vi "SingleSpectrum.vi"(0 "identifier out":string, 1 "Acquisition mode":u16(ring)=1 items=["Single spectrum", "Multiple spectra"], 2 "DPP Configuration":T1, 3 "Number of boards in chain":u8(slide)=1 scale=1.0..8.0, 4 "Boards to configure":u8(slide) scale=0.0..8.0, 6 "Start acq":bool, 7 "Stop":bool, 9 "Map points":u32=10, 11 "Time per spectrum [ms]":u32=10 max=1000000, 12 "reference":refnum<vi>, 13 "Acquisition time [s]":dbl=10.0 min=0.0009999999310821295 max=1000.0, 17 "Waveform Refnum":refnum<vi>, 18 "LastSpectra Refnum":refnum<vi>, 19 "SpectraPlot Refnum":refnum<vi>) -> (10 "Error code":i32, 14 "Acq. in progress":bool, 15 "Waveform Graph":dbl[][](graph))   [LabVIEW 2015]
uses:
  SingleSpectrumAcq.ctl
  GlobalParameters/SpectraData2.vi
  XGL_DPP.lvlib
panel:
  out "final time":u32
  out "live time":u32
  out "Init time":u32
  out "total_time":u32
  out "spectra to read":i64=1
  out "Statistics":dbl[][](array[numeric])
  out "adv stats":u64[][](array[numeric])
  out "spectra":u16[][](array[numeric])
  out "Library Initialized":bool
  in  "IP Address":string="10.96.0.110"
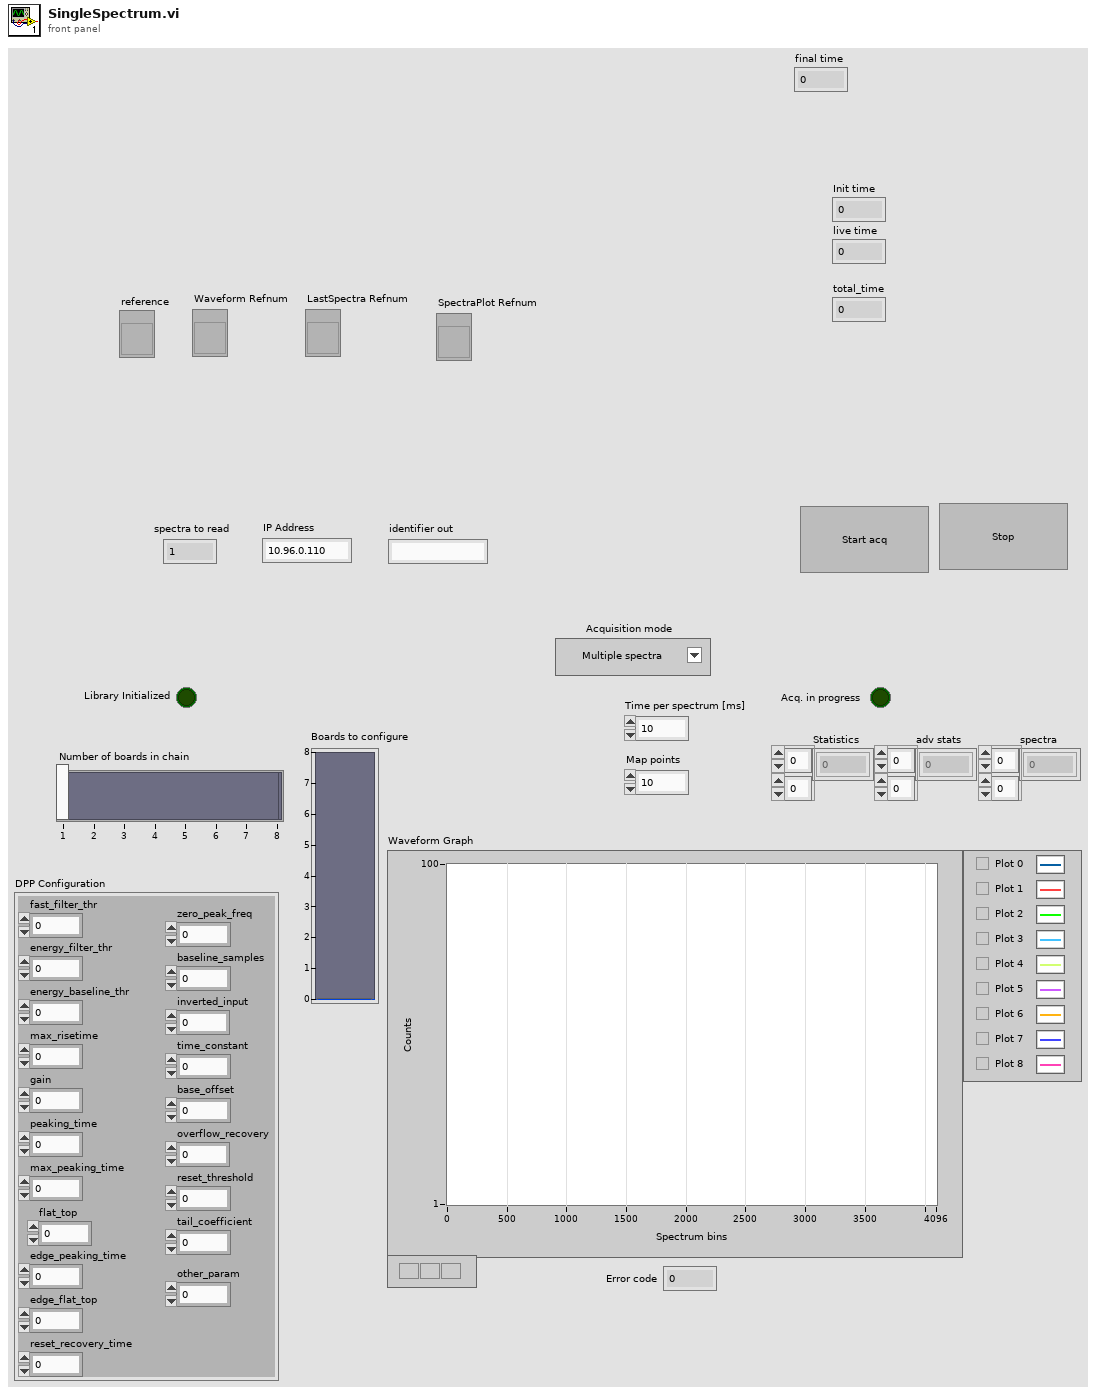
[diagram p1: front panel]
types:
  T1 = cluster{"reset_recovery_time":u32, "edge_peaking_time":u32, "flat_top":u32, "peaking_time":u32, "gain":dbl, "max_risetime":dbl, "fast_filter_thr":u32, "zero_peak_freq":dbl, "inverted_input":u8, "base_offset":u32, "reset_threshold":u32, "overflow_recovery":u32, "tail_coefficient":dbl, "energy_filter_thr":u32, "energy_baseline_thr":u32, "max_peaking_time":u32, "edge_flat_top":u32, "time_constant":dbl, "baseline_samples":u32, "other_param":u32}
  T2 = typedef "SingleSpectrumAcq.ctl" = enum16{"Stop", "Check downloaded spectra", "Get all data", "Read acq mode", "Send running/Get Data", "Clear", "Acquisition start", "Check Answer", "Wait Answer", "Start map"}
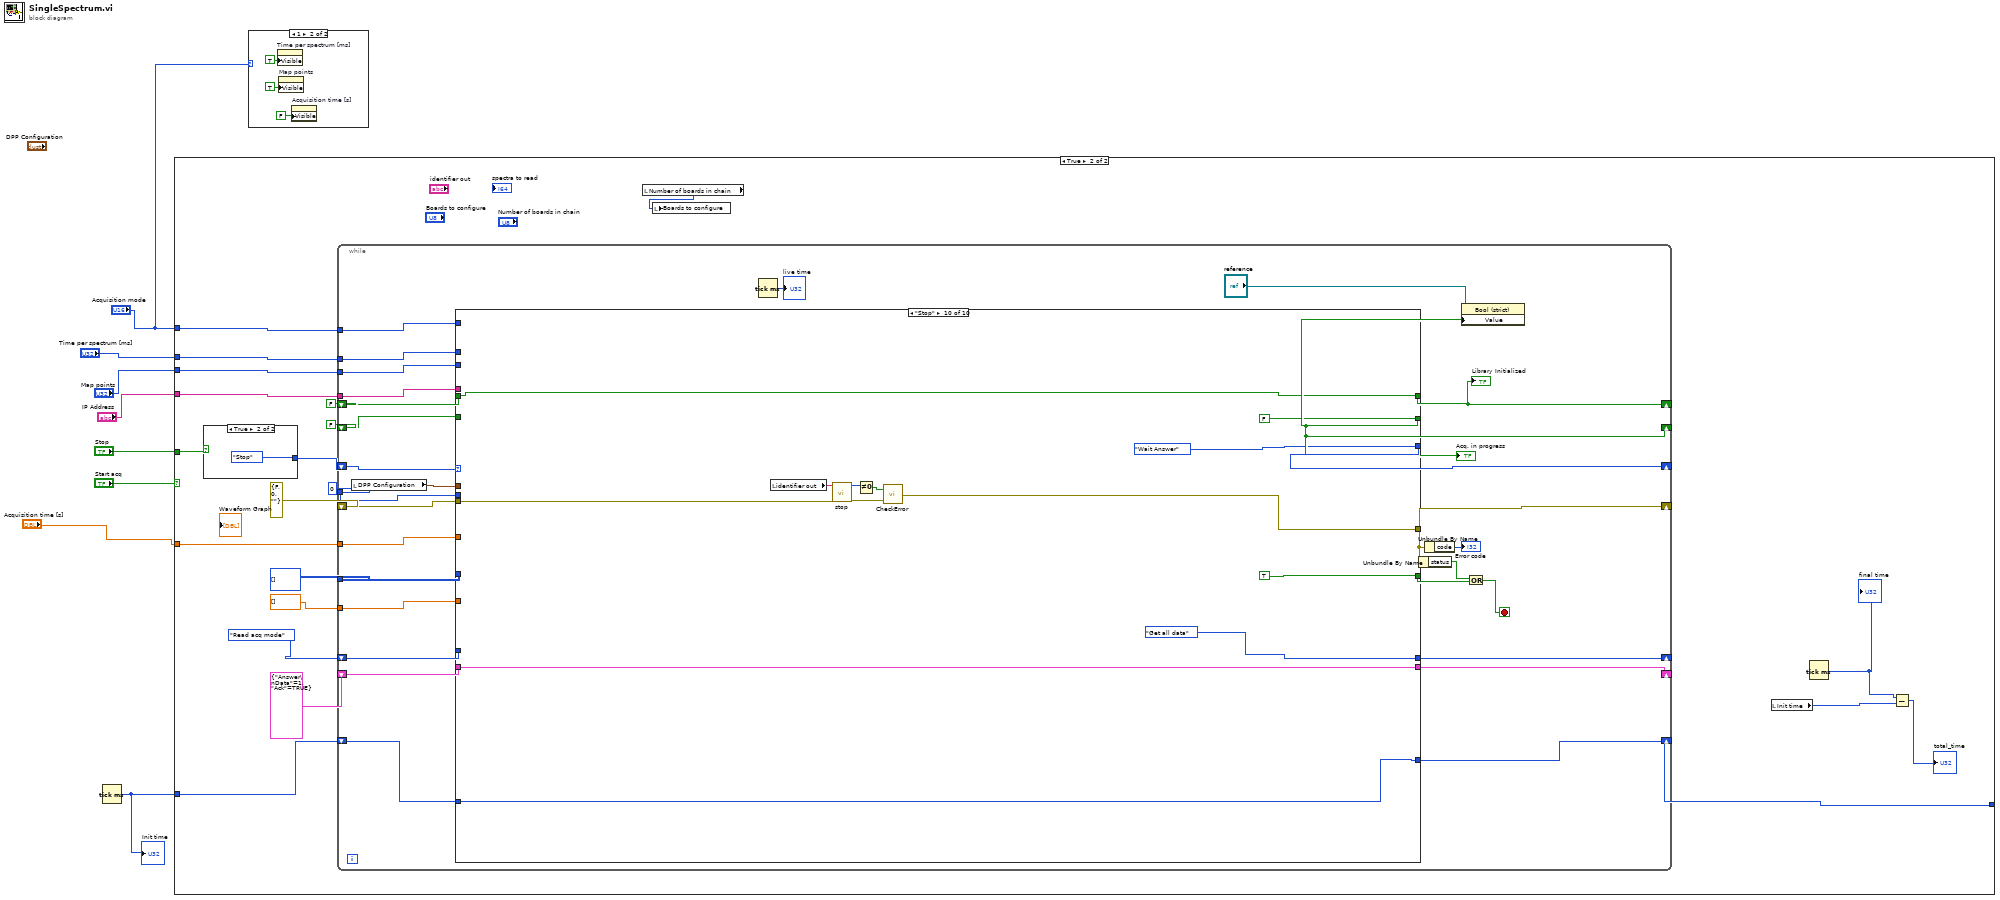
[diagram p0: block diagram]
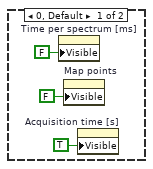
[diagram p2: hidden frame]
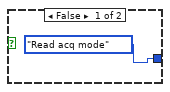
[diagram p4: hidden frame]
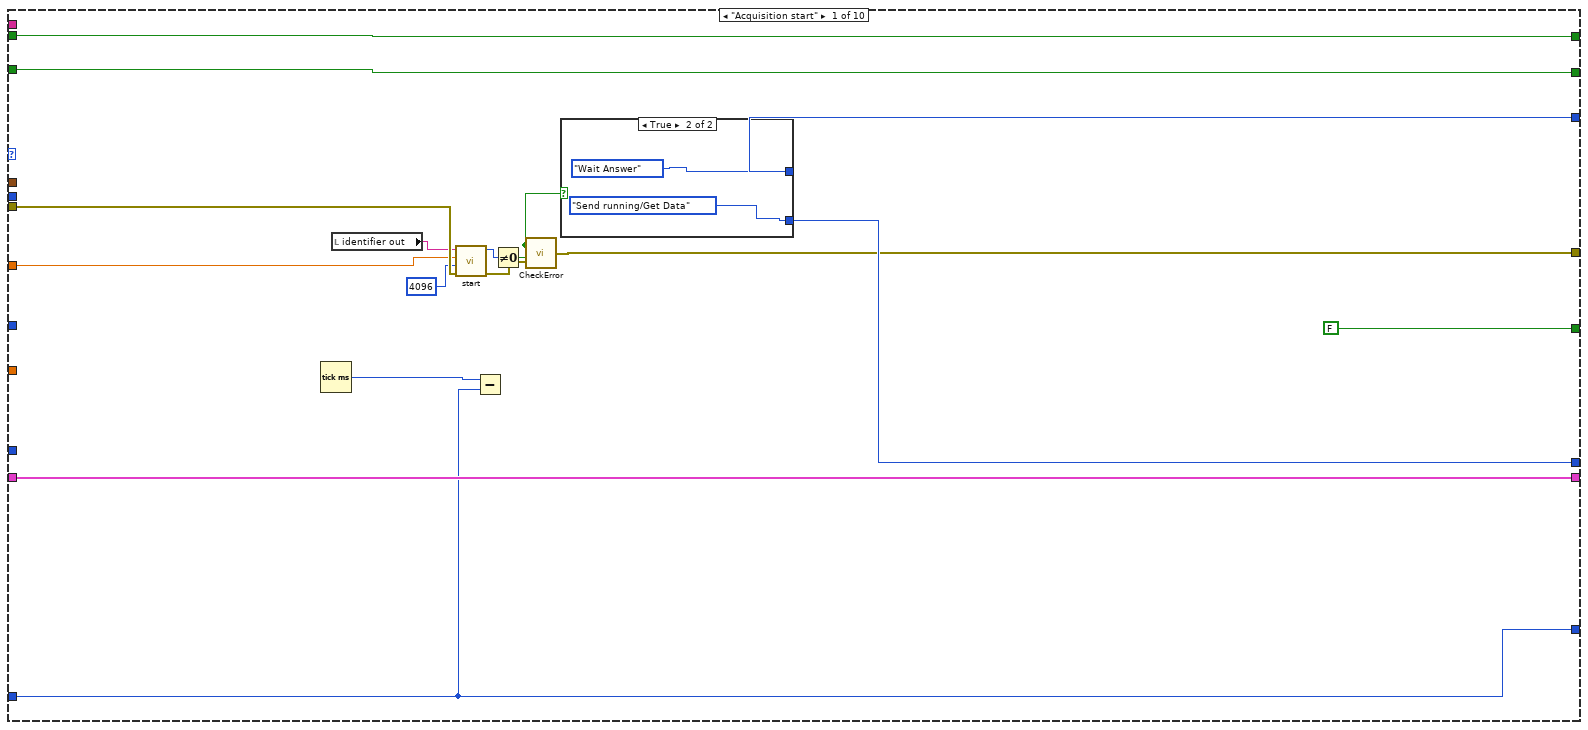
[diagram p5: hidden frame]
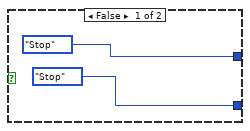
[diagram p6: hidden frame]
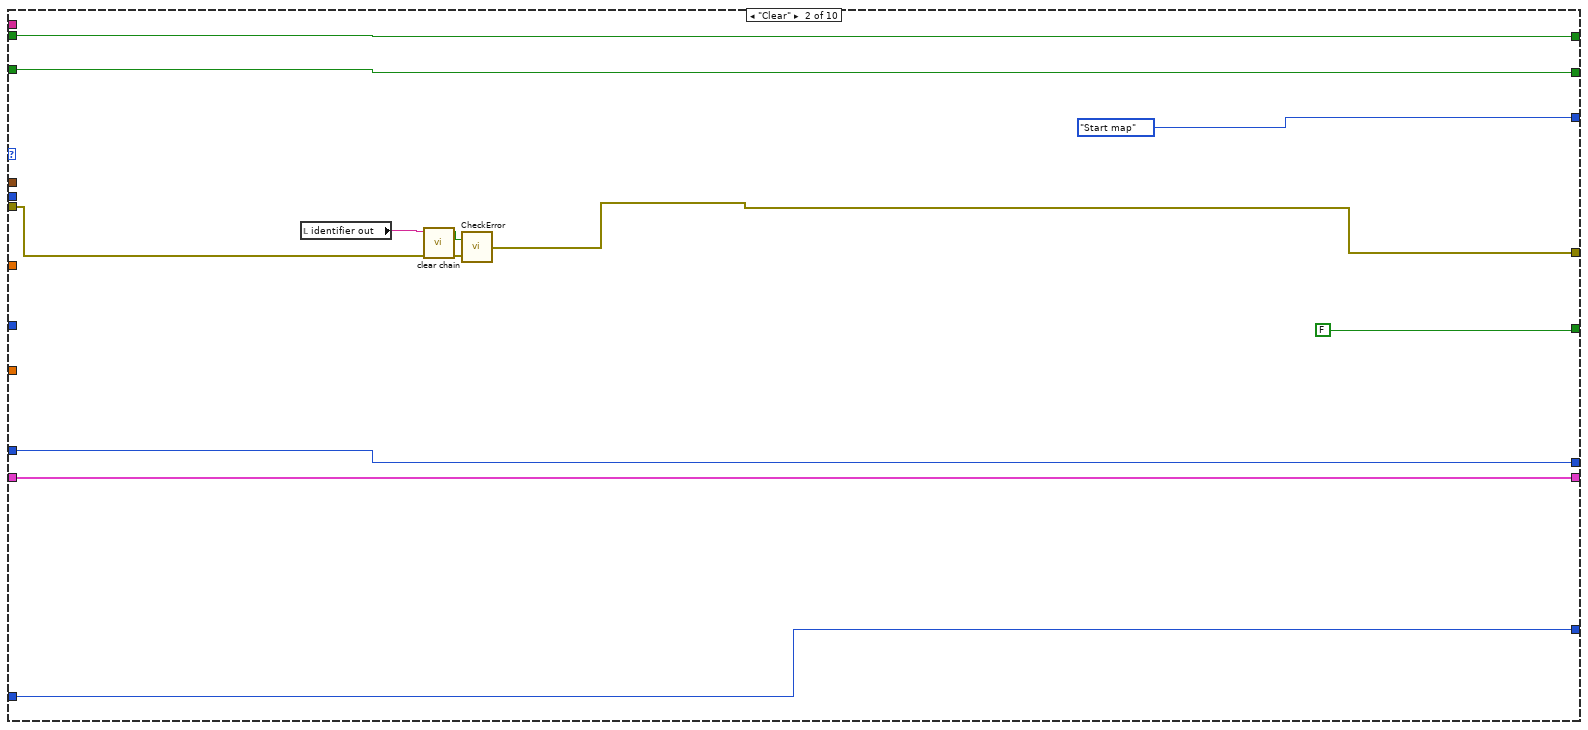
[diagram p7: hidden frame]
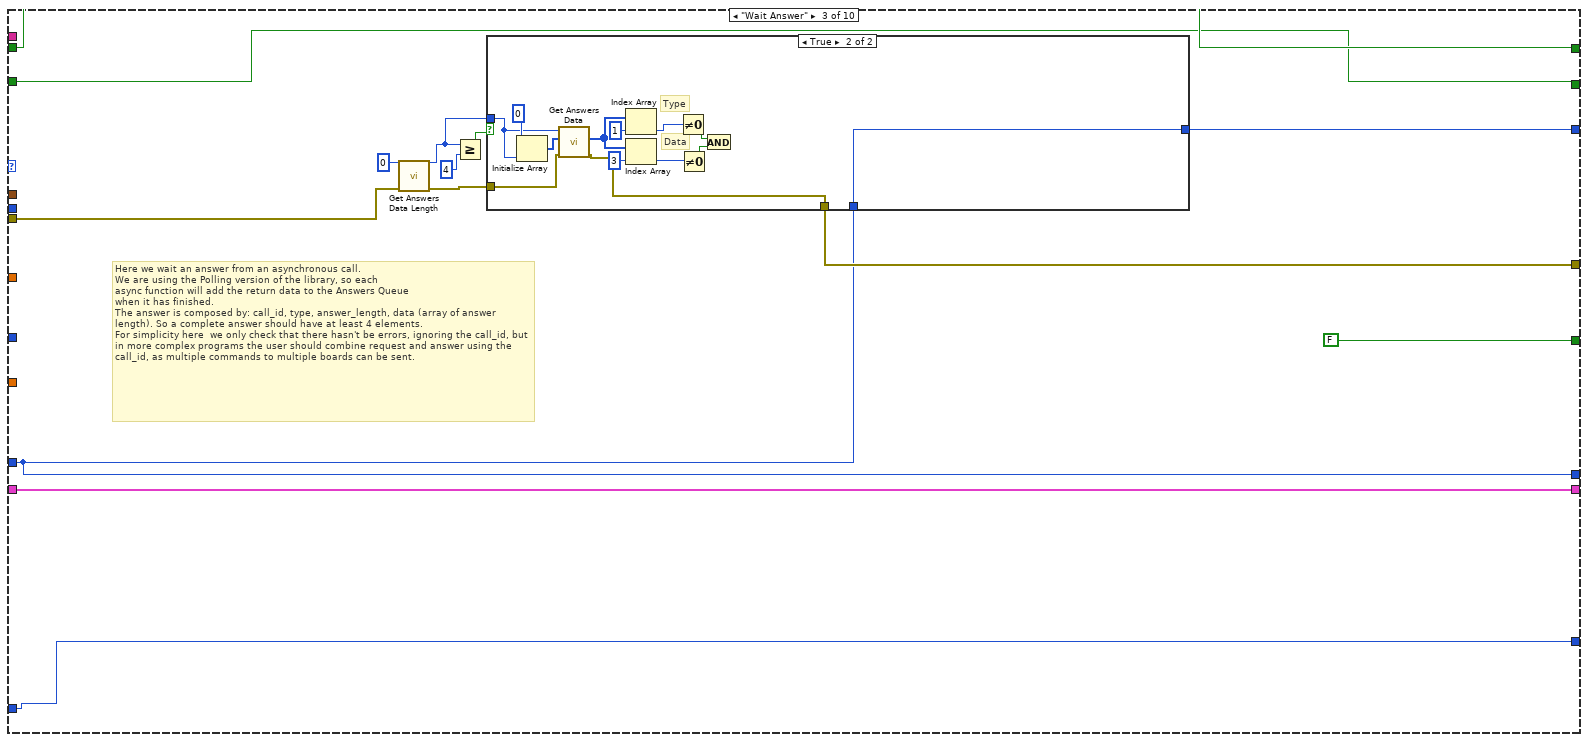
[diagram p8: hidden frame]
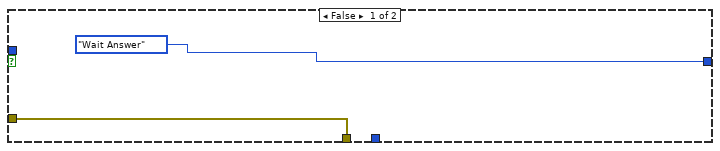
[diagram p9: hidden frame]
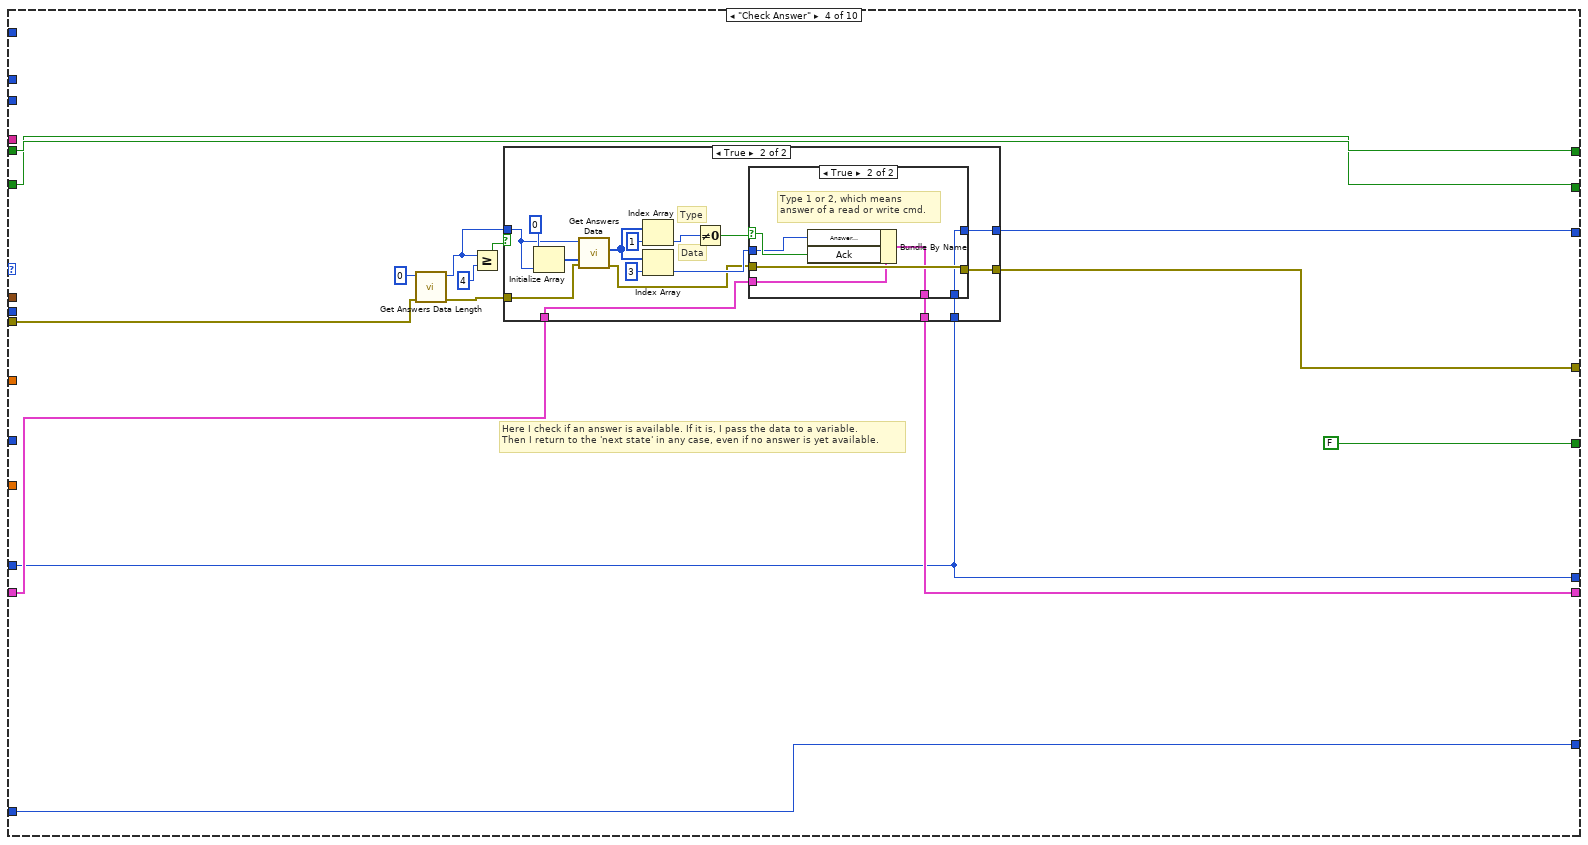
[diagram p10: hidden frame]
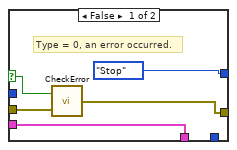
[diagram p12: hidden frame]
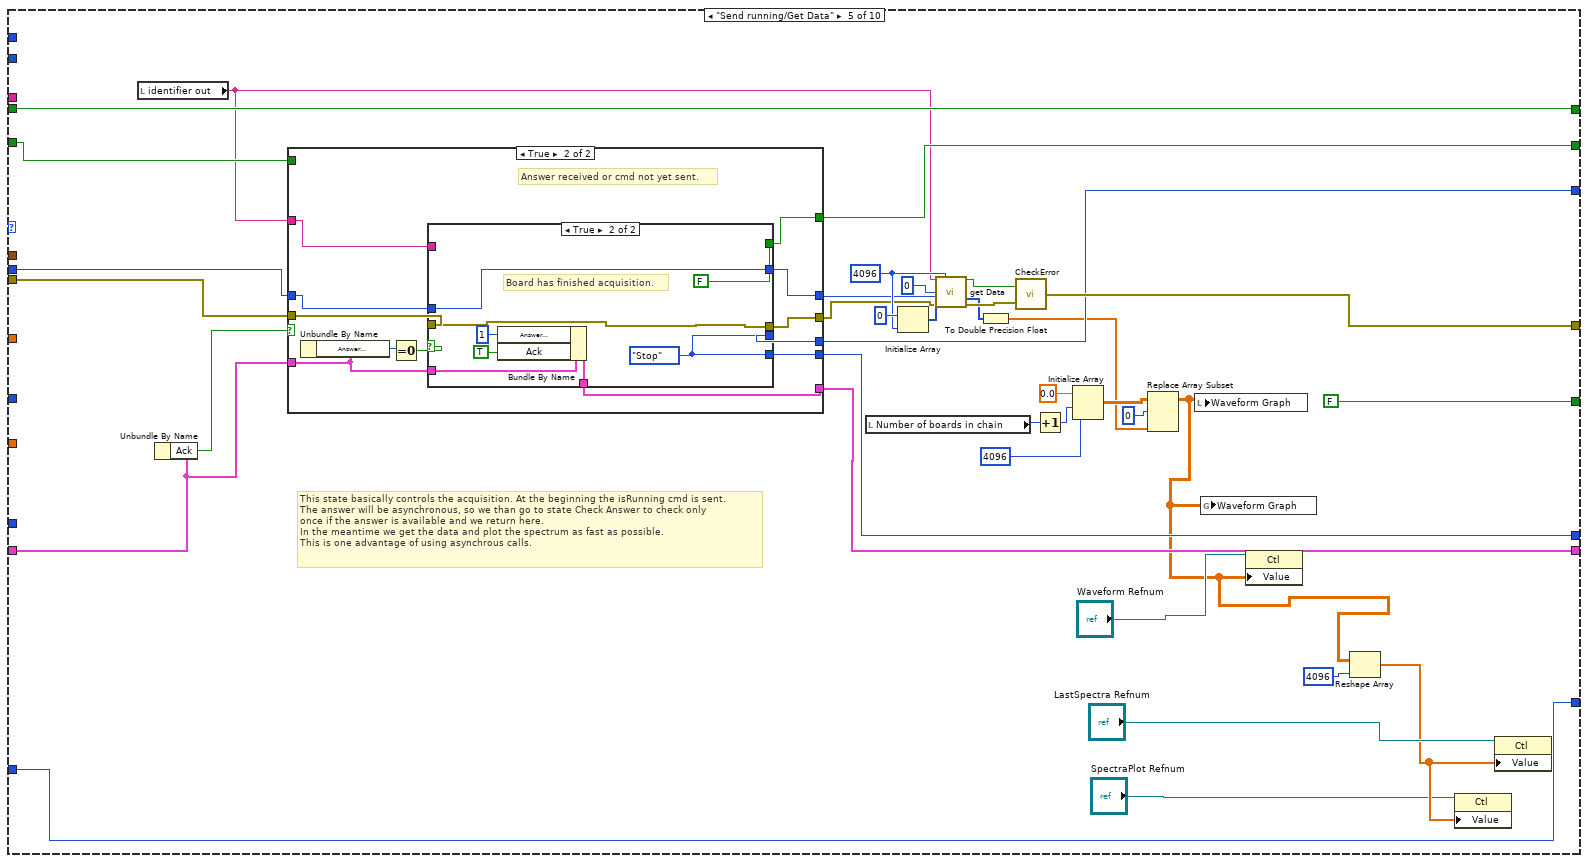
[diagram p13: hidden frame]
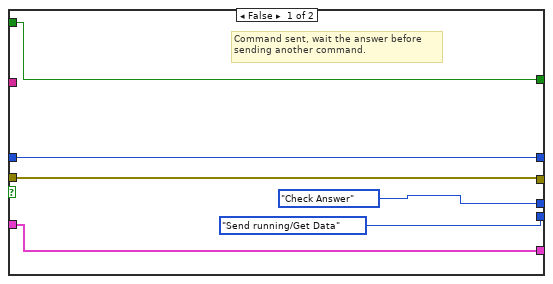
[diagram p14: hidden frame]
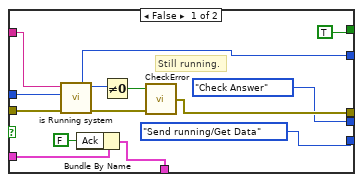
[diagram p15: hidden frame]
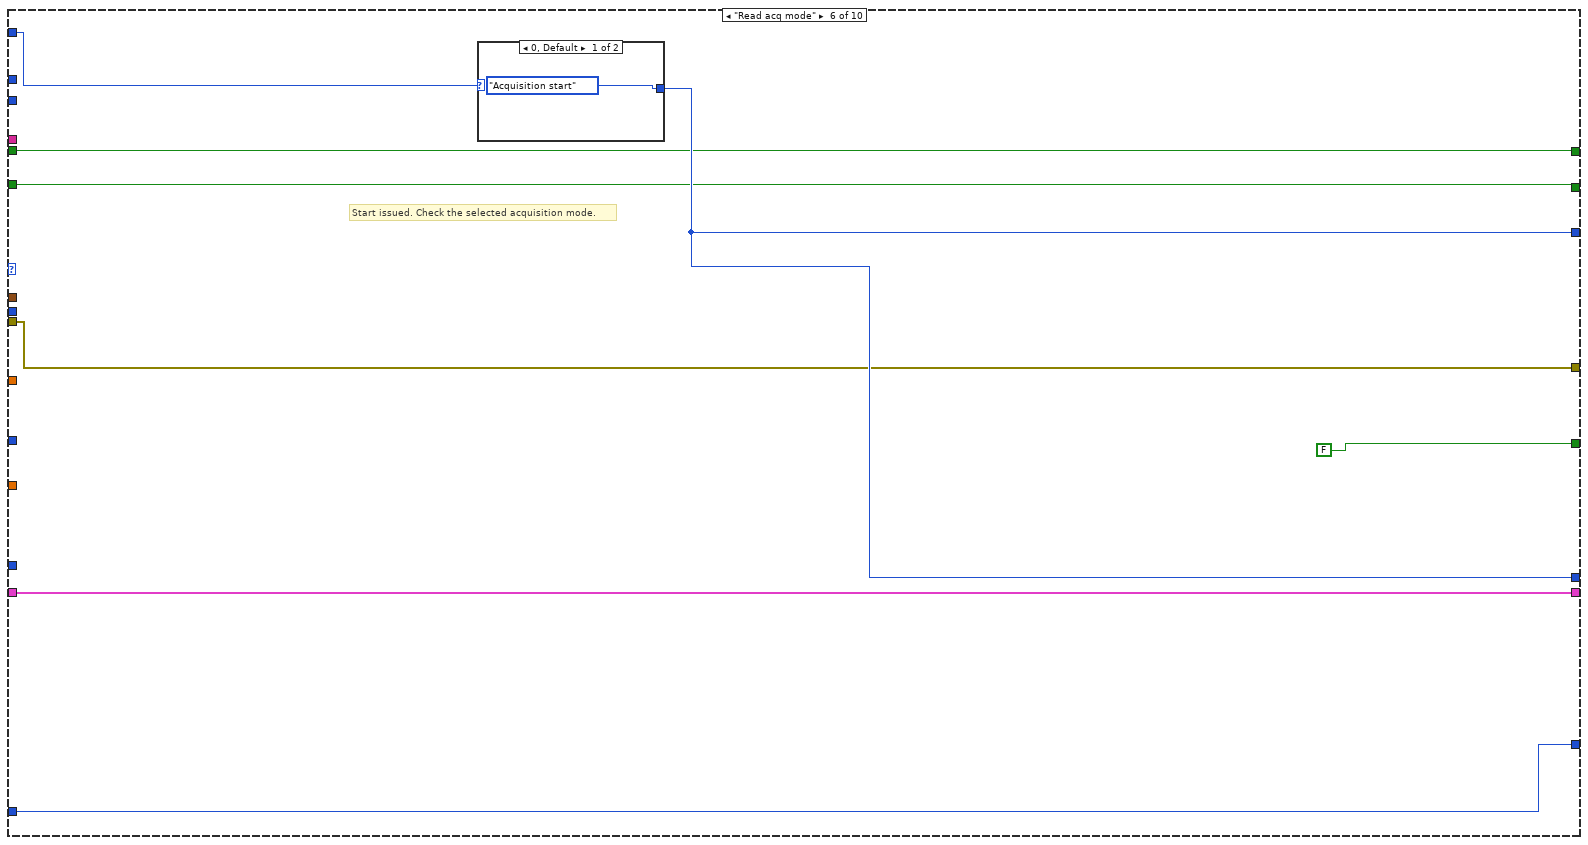
[diagram p16: hidden frame]
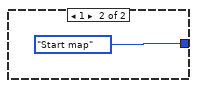
[diagram p17: hidden frame]
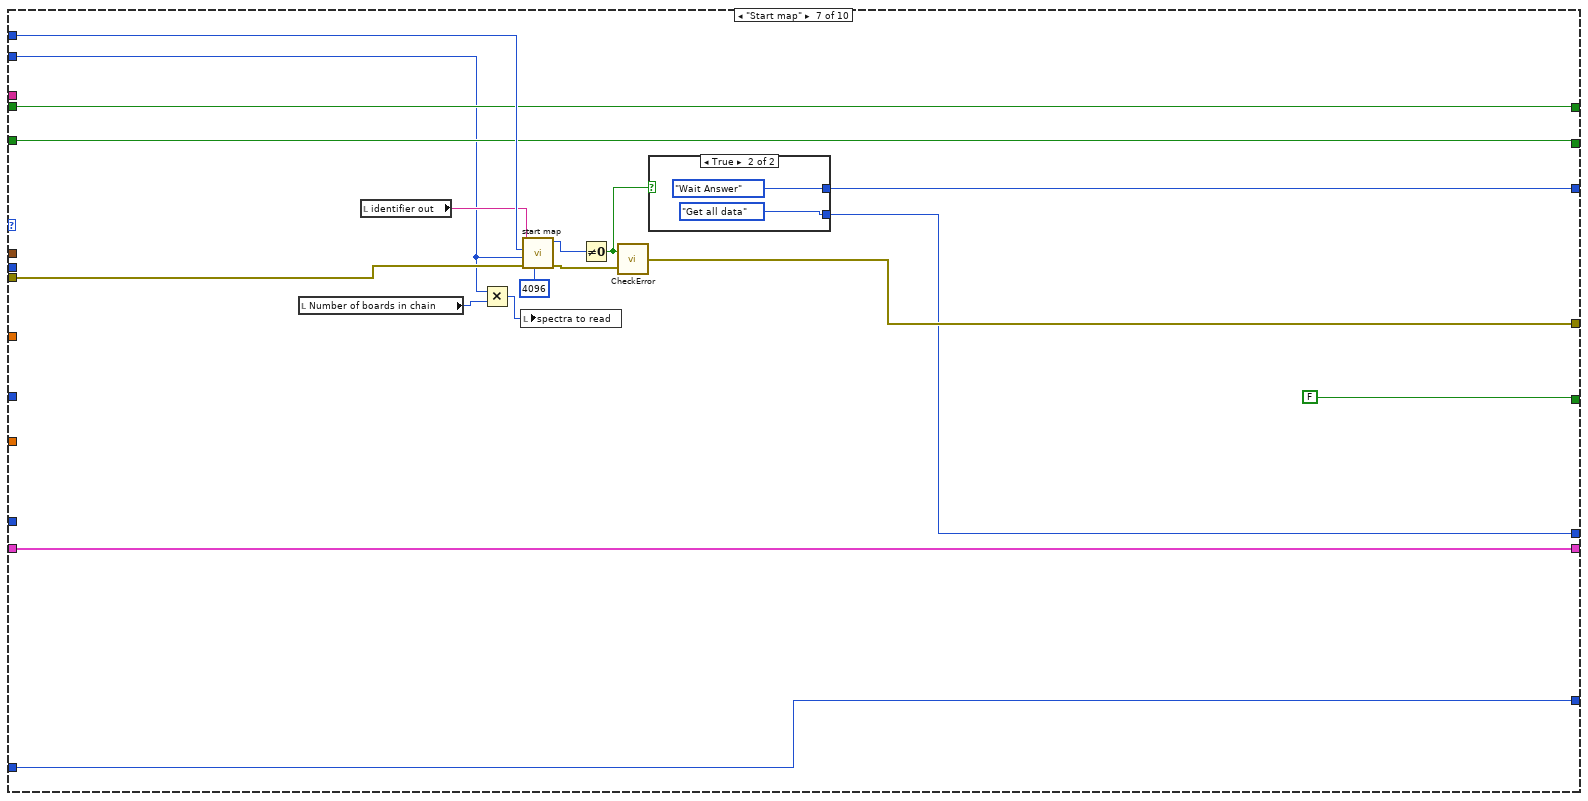
[diagram p18: hidden frame]
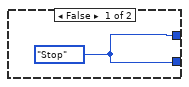
[diagram p19: hidden frame]
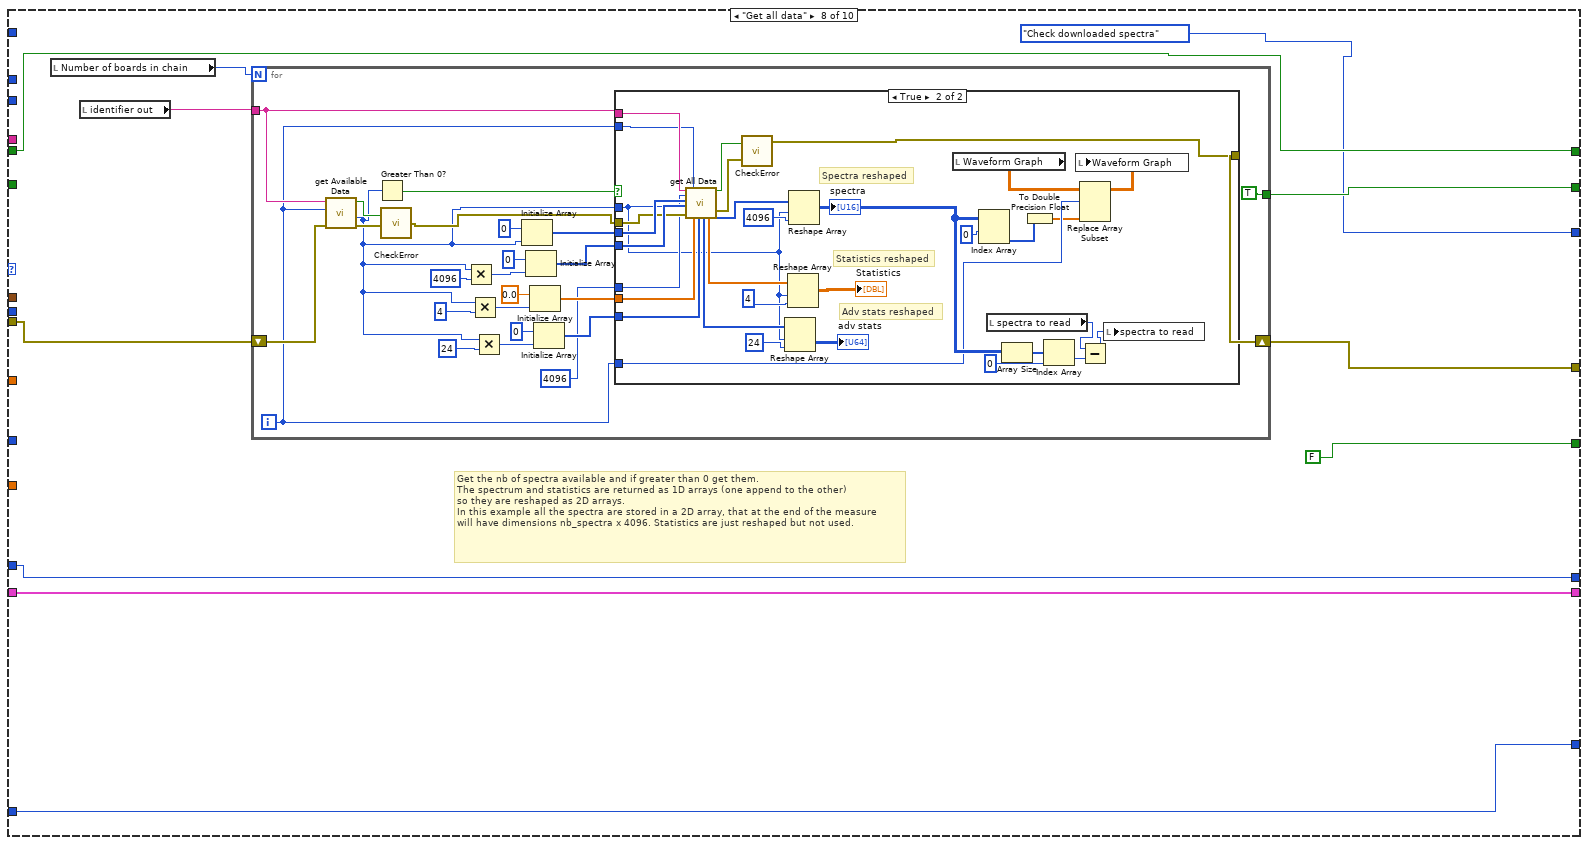
[diagram p20: hidden frame]
diagram:
  n1 = Tick Count (ms)() -> (millisecond timer value=w2:u32)
  "Init time" <- w2
  n2 = case shown="True" "Start acq" {
    tunnel: "Acquisition mode" -> [_ w21]
    tunnel: "Time per spectrum [ms]" -> [_ w20]
    tunnel: "Map points" -> [_ w19]
    tunnel: "IP Address" -> [_ w18]
    tunnel: "Acquisition time [s]" -> [_ w17]
    tunnel: "Stop" -> [_ w16]
    tunnel: w2 -> [w9 w14]
    tunnel: [w9 w13] -> _
    frame False {
    }
    frame True {
      n3 = case shown="True" w16 {
        tunnel: [SingleSpectrumAcq."Read acq mode" ("State") SingleSpectrumAcq."Stop" ("State")] -> w15
        frame False {
        }
        frame True {
        }
      }
      n4 = while {
        shift-right: [w59] -> _
        shift-left: errorcluster {"status"=FALSE, "code"=0, "source"=""} ("error in (no error)") -> [w61]
        shift-right: [w49] -> _
        shift-left: w15 -> [w46]
        shift-right: [w54] -> _
        shift-left: FALSE -> [w55]
        shift-right: [w38] -> _
        shift-left: FALSE -> [w53]
        tunnel: u16 0 ("Board") -> [w52]
        shift-right: [w51] -> _
        shift-left: SingleSpectrumAcq."Read acq mode" ("State") -> [w50]
        shift-right: [w47] -> _
        shift-left: cluster{"Answer\nData":i32, "Ack":bool} {"Answer\nData"=1, "Ack"=TRUE} -> [w48]
        tunnel: dbl[] [] ("Y") -> [w45]
        tunnel: u16[][] [] ("element") -> [w44]
        tunnel: w21 -> [w43]
        tunnel: w20 -> [w42]
        tunnel: w19 -> [w41]
        tunnel: w18 -> [w40]
        tunnel: w17 -> [w39]
        shift-right: [w34] -> w13
        shift-left: w14 -> [w35]
        stop <- w58 stop-if-true
        n5 = local read "DPP Configuration"() -> (w36:T1)
        n6 = case shown="\"Stop\"" w46 {
          tunnel: w61 -> [w75 w88 w107 w131 w202 w246 w268 w279 w355 w382]
          tunnel: [w69 w83 w101 w130 w193 w246 w265 w277 w355 w378] -> w59
          tunnel: [w73 SingleSpectrumAcq."Start map" ("State") w97 w129 w187 w249 w264 SingleSpectrumAcq."Check downloaded spectra" ("State") w357 SingleSpectrumAcq."Wait Answer" ("State")] -> w49
          tunnel: w39 -> [w74 _ _ _ _ _ _ _ _ _]
          tunnel: [FALSE ("y") FALSE ("y") FALSE ("y") FALSE ("y") FALSE ("y") FALSE FALSE FALSE FALSE TRUE] -> w56
          tunnel: [w77 w92 w99 w125 w191 w248 w262 w281 w356 w375] -> w54
          tunnel: w55 -> [w77 w92 w99 w125 w191 w248 w262 w281 w356 w375]
          tunnel: [w76 w91 w98 w124 w185 w247 w261 w282 w344 FALSE] -> w38
          tunnel: w53 -> [w76 w91 w98 w124 w184 w247 w261 _ _ _]
          tunnel: w52 -> [_ _ _ _ w203 _ _ _ _ _]
          tunnel: [w71 w90 w94 w126 w188 w249 w263 w283 w353 SingleSpectrumAcq."Get all data" ("State")] -> w51
          tunnel: w50 -> [_ w90 w94 w126 _ _ _ w283 w353 _]
          tunnel: w40 -> [_ _ _ _ _ _ _ _ _ _]
          tunnel: w36 -> [_ _ _ _ _ _ _ _ _ _]
          tunnel: w48 -> [w68 w89 w96 w128 w190 w244 w259 w284 w352 w377]
          tunnel: [w68 w89 w96 w127 w189 w244 w259 w284 w352 w377] -> w47
          tunnel: w43 -> [_ _ _ _ _ w250 _ _ _ _]
          tunnel: w42 -> [_ _ _ _ _ _ w269 _ w351 _]
          tunnel: w41 -> [_ _ _ _ _ _ w256 _ _ _]
          tunnel: w44 -> [_ _ _ _ _ _ _ _ _ _]
          tunnel: w45 -> [_ _ _ _ _ _ _ _ _ _]
          tunnel: w35 -> [w62 w82 w95 w123 w169 w243 w253 w274 w343 w370]
          tunnel: [w62 w82 w95 w123 w169 w243 w253 w274 w343 w370] -> w34
          frame "Acquisition start" {
            n7 = Tick Count (ms)() -> (millisecond timer value=w63:u32)
            n8 = local read "identifier out"() -> (w65:string)
            n9 = call "start.vi"("error in (no error)"=w75, "spect_depth"=u16 4096, "time"=w74, "identifier"=w65) -> ("error out"=w70:errorcluster, "function return"=w67:u32)  [unwired: 6 in]
            n10 = Subtract(x=w63, y=w62) -> ()  [unwired: 1 out]
            n11 = Not Equal To 0?(x=w67) -> (x != 0?=w66:bool)
            n12 = call "CheckError.vi"("error in (no error)"=w70, "ret_val"=w66) -> ("error out"=w69:errorcluster)
            n13 = case shown="True" w66 {
              tunnel: [SingleSpectrumAcq."Stop" ("State") SingleSpectrumAcq."Wait Answer" ("State")] -> w73
              tunnel: [SingleSpectrumAcq."Stop" ("State") SingleSpectrumAcq."Send running/Get Data" ("State")] -> w71
              frame False {
              }
              frame True {
              }
            }
          }
          frame "Clear" {
            n14 = local read "identifier out"() -> (w85:string)
            n15 = call "clear chain.vi"("error in (no error)"=w88, "identifier"=w85) -> ("error out"=w86:errorcluster, "function return"=w87:bool)  [unwired: 8 in]
            n16 = call "CheckError.vi"("error in (no error)"=w86, "ret_val"=w87) -> ("error out"=w83:errorcluster)
          }
          frame "Wait Answer" {
            # "Here we wait an answer from an asynchronous call.\nWe are using the Polling version of the library, so each\nasync function will add the return data to the Answers Queue\nwhen it has finished.\nThe answer is composed by: call_id, type, answer_length, data (array of answer length). So a complete answer should have at least 4 elements.\nFor simplicity here  we only check that there hasn't be errors, ignoring the call_id, but in more complex programs the user should combine request and answer using the call_id, as multiple commands to multiple boards can be sent."
            n17 = call "Get Answers Data Length.vi"("error in (no error)"=w107, "length"=u32 0) -> ("error out"=w103:errorcluster, "length out"=w102:u32)  [unwired: 7 in, 1 out]
            n18 = Greater Or Equal?(x=w102, y=u32 4) -> (x >= y?=w104:bool)
            n19 = case shown="True" w104 {
              tunnel: w103 -> [w109 w113]
              tunnel: w102 -> [_ w115]
              tunnel: [w109 w112] -> w101
              tunnel: [SingleSpectrumAcq."Wait Answer" ("State") w110] -> w97
              tunnel: w94 -> [_ w110]
              frame False {
              }
              frame True {
                # "Data"
                # "Type"
                n20 = Initialize Array(u32 0 ("y"), w115) -> (w114:u32[])
                n21 = call "Get Answers Data.vi"("error in (no error)"=w113, "data"=w114, "length"=w115) -> ("error out"=w112:errorcluster, "data out"=w111:u32[])  [unwired: 4 in, 1 out]
                n22 = Index Array(array=w111, index=1) -> (element=w118:u32)
                n23 = Index Array(array=w111, index=3) -> (element=w119:u32)
                n24 = Not Equal To 0?(x=w118) -> (x != 0?=w116:bool)
                n25 = Not Equal To 0?(x=w119) -> (x != 0?=w117:bool)
                n26 = And(x=w116, y=w117) -> ()  [unwired: 1 out]
              }
            }
          }
          frame "Check Answer" {
            # "Here I check if an answer is available. If it is, I pass the data to a variable.\nThen I return to the 'next state' in any case, even if no answer is yet available."
            n27 = call "Get Answers Data Length.vi"("error in (no error)"=w131, "length"=u32 0) -> ("error out"=w133:errorcluster, "length out"=w132:u32)  [unwired: 7 in, 1 out]
            n28 = Greater Or Equal?(x=w132, y=u32 4) -> (x >= y?=w134:bool)
            n29 = case shown="True" w134 {
              tunnel: w133 -> [w140 w145]
              tunnel: w132 -> [_ w143]
              tunnel: [w140 w151] -> w130
              tunnel: [w139 w150] -> w129
              tunnel: w126 -> [w139 w149]
              tunnel: w128 -> [w138 w147]
              tunnel: [w138 w148] -> w127
              frame False {
                # "Do not update answer data."
              }
              frame True {
                # "Data"
                # "Type"
                n30 = Initialize Array(u32 0 ("y"), w143) -> (w142:u32[])
                n31 = call "Get Answers Data.vi"("error in (no error)"=w145, "data"=w142, "length"=w143) -> ("error out"=w144:errorcluster, "data out"=w141:u32[])  [unwired: 4 in, 1 out]
                n32 = Index Array(array=w141, index=1) -> (element=w153:u32)
                n33 = Index Array(array=w141, index=3) -> (element=w146:u32)
                n34 = Not Equal To 0?(x=w153) -> (x != 0?=w152:bool)
                n35 = case shown="True" w152 {
                  selector: w152 -> [w161 w163]
                  tunnel: w144 -> [w160 w167]
                  tunnel: [w159 w167] -> w151
                  tunnel: [SingleSpectrumAcq."Stop" ("State") w166] -> w150
                  tunnel: w149 -> [_ w166]
                  tunnel: [w158 w164] -> w148
                  tunnel: w147 -> [w158 w165]
                  tunnel: w146 -> [_ w162]
                  frame False {
                    # "Type = 0, an error occurred."
                    n36 = call "CheckError.vi"("error in (no error)"=w160, "ret_val"=w161) -> ("error out"=w159:errorcluster)
                  }
                  frame True {
                    # "Type 1 or 2, which means\nanswer of a read or write cmd."
                    n37 = Bundle By Name(cluster=w165, "Answer\nData"=w162, "Ack"=w163) -> (w164:cluster{"Answer\nData":i32, "Ack":bool})
                  }
                }
              }
            }
          }
          frame "Send running/Get Data" {
            w198 = u32 4096 ("spectra_size")
            # "This state basically controls the acquisition. At the beginning the isRunning cmd is sent.\nThe answer will be asynchronous, so we than go to state Check Answer to check only\nonce if the answer is available and we return here.\nIn the meantime we get the data and plot the spectrum as fast as possible.\nThis is one advantage of using asynchrous calls."
            n38 = local read "identifier out"() -> (w183:string)
            n39 = Unbundle By Name(w190) -> ("Ack"=w201:bool)
            n40 = case shown="True" w201 {
              tunnel: w203 -> [w209 w216]
              tunnel: w202 -> [w208 w217]
              tunnel: [w208 w215] -> w194
              tunnel: [w209 w214] -> w192
              tunnel: w190 -> [w207 w219]
              tunnel: [w207 w218] -> w189
              tunnel: [SingleSpectrumAcq."Send running/Get Data" ("State") w213] -> w188
              tunnel: [SingleSpectrumAcq."Check Answer" ("State") w212] -> w187
              tunnel: [w206 w211] -> w185
              tunnel: w184 -> [w206 _]
              tunnel: w183 -> [_ w210]
              frame False {
                # "Command sent, wait the answer before\nsending another command."
              }
              frame True {
                # "Answer received or cmd not yet sent."
                n41 = Unbundle By Name(w219) -> ("Answer\nData"=w221:i32)
                n42 = Equal To 0?(x=w221) -> (x = 0?=w220:bool)
                n43 = case shown="True" w220 {
                  tunnel: [SingleSpectrumAcq."Send running/Get Data" ("State") w235] -> w213
                  tunnel: [SingleSpectrumAcq."Check Answer" ("State") w235] -> w212
                  tunnel: w219 -> [w231 w242]
                  tunnel: [w230 w239] -> w218
                  tunnel: w217 -> [w234 w237]
                  tunnel: w216 -> [w228 w238]
                  tunnel: [w232 w237] -> w215
                  tunnel: [w228 w238] -> w214
                  tunnel: [TRUE FALSE] -> w211
                  tunnel: w210 -> [w224 _]
                  frame False {
                    # "Still running."
                    n44 = call "is Running system.vi"("error in (no error)"=w234, "Board"=w228, "identifier"=w224) -> ("error out"=w233:errorcluster, "function return"=w225:u32)  [unwired: 7 in]
                    n45 = Bundle By Name(cluster=w231, "Ack"=FALSE) -> (w230:cluster{"Answer\nData":i32, "Ack":bool})
                    n46 = Not Equal To 0?(x=w225) -> (x != 0?=w226:bool)
                    n47 = call "CheckError.vi"("error in (no error)"=w233, "ret_val"=w226) -> ("error out"=w232:errorcluster)
                  }
                  frame True {
                    w235 = SingleSpectrumAcq."Stop" ("State")
                    # "Board has finished acquisition."
                    n48 = Bundle By Name(cluster=w242, "Answer\nData"=1 ("Answer\nData"), "Ack"=TRUE) -> (w239:cluster{"Answer\nData":i32, "Ack":bool})
                  }
                }
              }
            }
            n49 = local read "Number of boards in chain"() -> (w180:u8)
            n50 = Initialize Array(u64 0 ("acq_status"), w198) -> (w197:u64[])
            n51 = call "get Data.vi"("identifier"=w183, "spectra_size"=w198, "Board"=w192, "id"=u32 0, "values"=w197, "error in (no error)"=w194) -> ("function return"=w195:bool, "values out"=w182:u64[], "error out"=w196:errorcluster)  [unwired: 5 in, 2 out]
            n52 = To Double Precision Float(number=w182) -> (double precision float=w178:dbl[])
            n53 = call "CheckError.vi"("error in (no error)"=w196, "ret_val"=w195) -> ("error out"=w193:errorcluster)
            n54 = Increment(x=w180) -> (x+1=w176:u8)
            n55 = Initialize Array(0.0, w176, 4096 ("dimension size")) -> (w179:dbl[][])
            n56 = Replace Array Subset(array=w179, new element=w178, index (row)=0 ("disabled index (col)")) -> (w168:dbl[][])  [unwired: 1 in]
            n57 = local write "Waveform Graph"(w168) -> ()
            n58 = global write "SpectraData2.vi" "Waveform Graph"(w168) -> ()
            n59 = property on="Property Node" class="Ctl"(reference="Waveform Refnum", "Value"=w168) -> ()  [unwired: 1 in, 2 out]
            n60 = Reshape Array(w168, 4096 ("dimension size")) -> (w171:dbl[])
            n61 = property on="Property Node" class="Ctl"(reference="SpectraPlot Refnum", "Value"=w171) -> ()  [unwired: 1 in, 2 out]
            n62 = property on="Property Node" class="Ctl"(reference="LastSpectra Refnum", "Value"=w171) -> ()  [unwired: 1 in, 2 out]
          }
          frame "Read acq mode" {
            # "Start issued. Check the selected acquisition mode."
            n63 = case shown="0, Default" w250 {
              tunnel: [SingleSpectrumAcq."Acquisition start" ("State") SingleSpectrumAcq."Start map" ("State")] -> w249
              frame 0, Default {
              }
              frame 1 {
              }
            }
          }
          frame "Start map" {
            n64 = local read "Number of boards in chain"() -> (w255:u8)
            n65 = local read "identifier out"() -> (w258:string)
            n66 = Multiply(x=w256, y=w255) -> (x*y=w257:u32)
            n67 = local write "spectra to read"(w257) -> ()
            n68 = call "start map.vi"("spect_depth"=u16 4096, "error in (no error)"=w268, "points"=w256, "sp_time"=w269, "identifier"=w258) -> ("error out"=w267:errorcluster, "function return"=w266:u32)  [unwired: 5 in]
            n69 = Not Equal To 0?(x=w266) -> (x != 0?=w270:bool)
            n70 = call "CheckError.vi"("error in (no error)"=w267, "ret_val"=w270) -> ("error out"=w265:errorcluster)
            n71 = case shown="True" w270 {
              tunnel: [w271 SingleSpectrumAcq."Wait Answer" ("State")] -> w264
              tunnel: [w271 SingleSpectrumAcq."Get all data" ("State")] -> w263
              frame False {
                w271 = SingleSpectrumAcq."Stop" ("State")
              }
              frame True {
              }
            }
          }
          frame "Get all data" {
            # "Get the nb of spectra available and if greater than 0 get them.\nThe spectrum and statistics are returned as 1D arrays (one append to the other)\nso they are reshaped as 2D arrays.\nIn this example all the spectra are stored in a 2D array, that at the end of the measure \nwill have dimensions nb_spectra x 4096. Statistics are just reshaped but not used."
            n72 = local read "Number of boards in chain"() -> (w276:u8)
            n73 = local read "identifier out"() -> (w278:string)
            n74 = for {
              N: w276 -> [_]
              tunnel: [TRUE] -> w282
              tunnel: w278 -> [w291]
              shift-right: [w286] -> w277
              shift-left: w279 -> [w293]
              i -> [w285]
              n75 = call "get Available Data.vi"("error in (no error)"=w293, "Board"=w285, "identifier"=w291) -> ("error out"=w308:errorcluster, "data_number out"=w294:u32, "function return"=w309:bool)  [unwired: 6 in]
              n76 = Greater Than 0?(x=w294) -> (x > 0?=w307:bool)
              n77 = call "CheckError.vi"("error in (no error)"=w308, "ret_val"=w309) -> ("error out"=w306:errorcluster)
              n78 = Multiply(x=w294, y=u32 4096) -> (x*y=w301:u32)
              n79 = Multiply(x=w294, y=u32 4) -> (x*y=w298:u32)
              n80 = Multiply(x=w294, y=u32 24) -> (x*y=w295:u32)
              n81 = Initialize Array(u32 0, w294) -> (w292:u32[])
              n82 = Initialize Array(u16 0, w301) -> (w290:u16[])
              n83 = Initialize Array(0.0, w298) -> (w289:dbl[])
              n84 = Initialize Array(u64 0, w295) -> (w288:u64[])
              n85 = case shown="True" w307 {
                tunnel: w285 -> [_ w322]
                tunnel: w306 -> [w310 w319]
                tunnel: [w310 w337] -> w286
                tunnel: w291 -> [_ w331]
                tunnel: w294 -> [_ w315]
                tunnel: w292 -> [_ w321]
                tunnel: w290 -> [_ w320]
                tunnel: u32 4096 ("spectra_size") -> [_ w318]
                tunnel: w289 -> [_ w317]
                tunnel: w288 -> [_ w316]
                tunnel: w285 -> [_ w312]
                frame False {
                  # "No spectrum available."
                }
                frame True {
                  # "Adv stats reshaped"
                  # "Statistics reshaped"
                  # "Spectra reshaped"
                  n86 = call "get All Data.vi"("identifier"=w331, "data_number"=w315, "id"=w321, "values"=w320, "error in (no error)"=w319, "spectra_size"=w318, "Board"=w322, "stats"=w317, "advstats"=w316) -> ("advstats out"=w340:u64[], "stats out"=w341:dbl[], "function return"=w339:bool, "values out"=w342:u16[], "error out"=w338:errorcluster)  [unwired: 3 in, 3 out]
                  n87 = call "CheckError.vi"("error in (no error)"=w338, "ret_val"=w339) -> ("error out"=w337:errorcluster)
                  n88 = Reshape Array(w340, w315, 24 ("dimension size")) -> (→"adv stats":u64[][])
                  n89 = Reshape Array(w341, w315, 4 ("dimension size")) -> (→"Statistics":dbl[][])
                  n90 = Reshape Array(w342, w315, u16 4096 ("dimension size")) -> (w328:u16[][])
                  "spectra" <- w328
                  n91 = local read "Waveform Graph"() -> (w313:dbl[][])
                  n92 = Index Array(array=w328, index (row)=0) -> (element=w333:u16[])  [unwired: 1 in]
                  n93 = local read "spectra to read"() -> (w325:i64)
                  n94 = Array Size(array=w328) -> (size(s)=w327:i32[])
                  n95 = To Double Precision Float(number=w333) -> (double precision float=w311:dbl[])
                  n96 = Index Array(array=w327, index=0) -> (element=w324:i32)
                  n97 = Replace Array Subset(array=w313, new element=w311, index (row)=w312) -> (w314:dbl[][])  [unwired: 1 in]
                  n98 = local write "Waveform Graph"(w314) -> ()
                  n99 = Subtract(x=w325, y=w324) -> (x-y=w323:i64)
                  n100 = local write "spectra to read"(w323) -> ()
                }
              }
            }
          }
          frame "Check downloaded spectra" {
            (unwired) dbl[][] []
            # "Check the current dimension of spectra 2D array. There can be this cases:\n- Downloaded spectra less than total_spectra-1 -> acquisition still in progress.\n- Down spectra equals total_spectra-1 ->acquisition almost finished, send stop.\nNote that the last spectrum will become available after the stop is sent. This because\nthe DLL mark as complete a spectrum if another spectrum arrives or the stop is issued.\n- Down spectra equals total_spectra -> acquisition finished, return to Wait Input."
            n101 = local read "Number of boards in chain"() -> (w345:u8)
            n102 = local read "spectra to read"() -> (w347:i64)
            n103 = Divide(x=w347, y=w345) -> (x/y=w346:dbl)
            n104 = Decrement(x=w346) -> (x-1=w350:dbl)
            n105 = Less Or Equal?(x=w350, y=u32 0) -> (x <= y?=w348:bool)
            n106 = case shown="True" w348 {
              tunnel: [SingleSpectrumAcq."Get all data" ("State") w364] -> w357
              tunnel: w351 -> [_ w363]
              tunnel: w350 -> [_ w362]
              tunnel: [TRUE w360] -> w344
              frame False {
              }
              frame True {
                n107 = Equal To 0?(x=w362) -> (x = 0?=w361:bool)
                n108 = case shown="True" w361 {
                  tunnel: [SingleSpectrumAcq."Stop" ("State") SingleSpectrumAcq."Stop" ("State")] -> w364
                  tunnel: w363 -> [w367 _]
                  tunnel: [TRUE FALSE] -> w360
                  frame True {
                    n109 = Wait (ms)(milliseconds to wait=w367) -> ()  [unwired: 1 out]
                  }
                  frame False {
                  }
                }
              }
            }
          }
          frame "Stop" {
            n110 = local read "identifier out"() -> (w373:string)
            n111 = call "stop.vi"("error in (no error)"=w382, "identifier"=w373) -> ("error out"=w379:errorcluster, "function return"=w381:u32)  [unwired: 8 in]
            n112 = Not Equal To 0?(x=w381) -> (x != 0?=w380:bool)
            n113 = call "CheckError.vi"("error in (no error)"=w379, "ret_val"=w380) -> ("error out"=w378:errorcluster)
          }
        }
        "Library Initialized" <- w54
        "Acq. in progress" <- w38
        n114 = Tick Count (ms)() -> (millisecond timer value=→"live time":u32)
        n115 = Unbundle By Name(w59) -> ("status"=w57:bool)
        n116 = Unbundle By Name(w59) -> ("code"=→"Error code":i32)
        n117 = property on="Property Node" class="Bool (strict)"(reference="reference", "Value"=w38) -> ()  [unwired: 1 in, 2 out]
        n118 = Or(x=w57, y=w56) -> (x .or. y?=w58:bool)
      }
      n119 = local read "Number of boards in chain"() -> (w22:u8)
      n120 = local write "Boards to configure"(w22) -> ()
      n121 = local read "Init time"() -> (w11:u32)
      n122 = Tick Count (ms)() -> (millisecond timer value=w10:u32)
      "final time" <- w10
      n123 = Subtract(x=w10, y=w11) -> (x-y=→"total_time":u32)
    }
  }
  n124 = case shown="1" "Acquisition mode" {
    frame 0, Default {
      n125 = property on="Time per spectrum [ms]" class="DigNum (strict)"("Visible"=FALSE) -> ()  [unwired: 2 in, 2 out]
      n126 = property on="Map points" class="DigNum (strict)"("Visible"=FALSE) -> ()  [unwired: 2 in, 2 out]
      n127 = property on="Acquisition time [s]" class="DigNum (strict)"("Visible"=TRUE) -> ()  [unwired: 2 in, 2 out]
    }
    frame 1 {
      n128 = property on="Time per spectrum [ms]" class="DigNum (strict)"("Visible"=TRUE) -> ()  [unwired: 2 in, 2 out]
      n129 = property on="Map points" class="DigNum (strict)"("Visible"=TRUE) -> ()  [unwired: 2 in, 2 out]
      n130 = property on="Acquisition time [s]" class="DigNum (strict)"("Visible"=FALSE) -> ()  [unwired: 2 in, 2 out]
    }
  }
